vi "aft_Simulate_Edit_Template_(LMS).vi"(6 "State In":T2, 8 "error in":errorcluster, 11 "Diagram":T1) -> (0 "error out":errorcluster)   [LabVIEW 2017, in "NI_AdaptiveFilter.lvlib"]
uses:
  <vilib>/addons/Adaptive Filters/NI_AdaptiveFilter.lvlib
  <vilib>/addons/Adaptive Filters/Fixed-Point Simulation/LMS/AFT Simulate Fixed-Point FIR LMS.ctl
  <vilib>/XNodeSupport/XNodeTopLevelDiagramRef.ctl
  <vilib>/fxp/LVFixedPointOverflowPolicyTypeDef.ctl
  <vilib>/fxp/LVFixedPointQuantizationPolicyTypeDef.ctl
  <vilib>/addons/Adaptive Filters/Fixed-Point Simulation/LMS/AFT Simulate Fixed-Point FIR LMS.xnode
  <vilib>/XNodeSupport/NI_XNodeSupport.lvlib
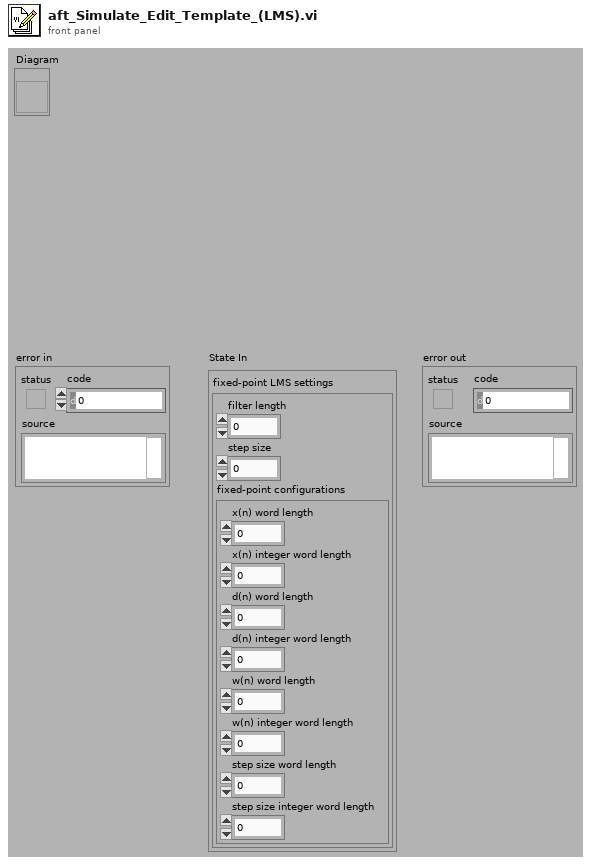
[diagram p1: front panel]
types:
  T1 = typedef "NI_XNodeSupport.lvlib/XNodeTopLevelDiagramRef.ctl" = refnum<vi>
  T2 = typedef "AFT Simulate Fixed-Point FIR LMS.xnode/AFT Simulate Fixed-Point FIR LMS.ctl" = cluster{"fixed-point LMS settings":cluster{"filter length":i32, "step size":dbl, "fixed-point configurations":cluster{"x(n) word length":i32, "x(n) integer word length":i32, "d(n) word length":i32, "d(n) integer word length":i32, "w(n) word length":i32, "w(n) integer word length":i32, "step size word length":i32, "step size integer word length":i32}}}
  T3 = typedef "LVFixedPointOverflowPolicyTypeDef.ctl" = enum32{"Wrap", "Saturate"}
  T4 = typedef "LVFixedPointQuantizationPolicyTypeDef.ctl" = enum32{"Truncate", "Round-Half-Up (Asymmetric)", "Round-Half-Even"}
  T5 = cluster{"filter length":i32, "step size":dbl, "fixed-point configurations":cluster{"x(n) word length":i32, "x(n) integer word length":i32, "d(n) word length":i32, "d(n) integer word length":i32, "w(n) word length":i32, "w(n) integer word length":i32, "step size word length":i32, "step size integer word length":i32}}
  T6 = cluster{"x(n) word length":i32, "x(n) integer word length":i32, "d(n) word length":i32, "d(n) integer word length":i32, "w(n) word length":i32, "w(n) integer word length":i32, "step size word length":i32, "step size integer word length":i32}
  T7 = typedef "LVFixedPointRepBitsTypeDef.ctl" = cluster{"Signed":bool, "Word Length":u32, "Integer Word Length":i32}
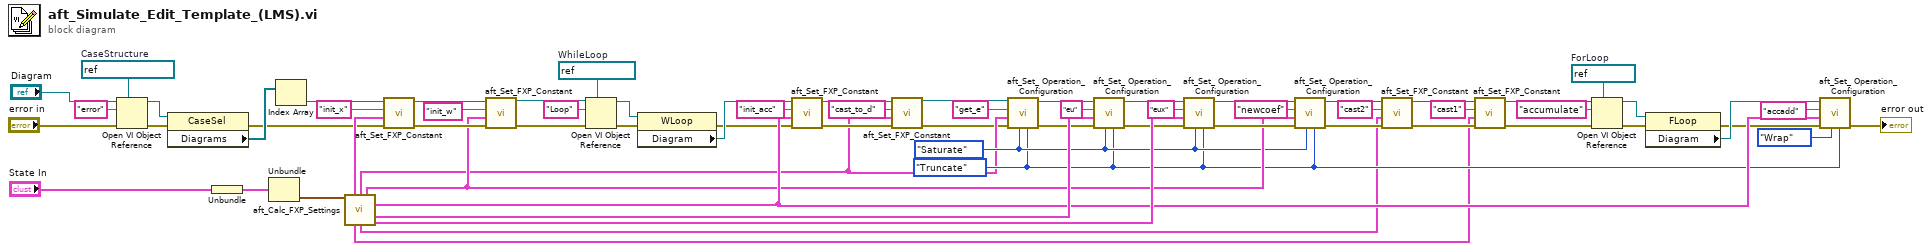
[diagram p0: block diagram]
diagram:
  w14 = LVFixedPointQuantizationPolicyTypeDef."Truncate" ("FXP Quantization Policy")
  w15 = LVFixedPointOverflowPolicyTypeDef."Saturate" ("FXP Overflow Policy")
  w43 = refnum<vi> refnum  # ForLoop
  w60 = refnum<vi> refnum  # WhileLoop
  w64 = refnum<vi> refnum  # CaseStructure
  n1 = Open VI Object Reference(7:w64, 8:"error in", 10:"error" ("name/order"), 11:"Diagram") -> (0:w19:errorcluster, 3:w58:refnum<vi>)
  n2 = property class="CaseSel"(reference=w58, error in=w19) -> (error out=w17:errorcluster, "Diagrams"=w62:refnum<vi>[])  [unwired: 1 out]
  n3 = Unbundle("State In") -> ("fixed-point LMS settings"=w66:T5)
  n4 = Unbundle(w66) -> ("fixed-point configurations"=w65:T6)  [unwired: 2 out]
  n5 = Index Array(array=w62) -> (element=w57:refnum<vi>)  [unwired: 1 in]
  n6 = call <vilib>:"aft_Calc_FXP_Settings.vi"("fixed-point configurations"=w65) -> ("x"=w27:T7, "d"=w12:T7, "w"=w20:T7, "init2"=w38:T7, "init3"=w49:T7, "cast 1"=w2:T7, "cast 2"=w1:T7, "init4"=w46:T7)  [unwired: 5 in, 2 out]
  n7 = call <vilib>:"aft_Set_FXP_Constant.vi"("error in (no error)"=w17, "fixed-point representation:bits"=w27, "name/order"="init_x", "diagram in"=w57) -> ("error out"=w25:errorcluster, "diagram out"=w23:refnum<vi>)  [unwired: 6 out]
  n8 = call <vilib>:"aft_Set_FXP_Constant.vi"("error in (no error)"=w25, "fixed-point representation:bits"=w20, "name/order"="init_w", "diagram in"=w23) -> ("error out"=w24:errorcluster, "diagram out"=w22:refnum<vi>)  [unwired: 6 out]
  n9 = Open VI Object Reference(7:w60, 8:w24, 10:"Loop" ("name/order"), 11:w22) -> (0:w37:errorcluster, 3:w56:refnum<vi>)
  n10 = property class="WLoop"(reference=w56, error in=w37) -> (error out=w36:errorcluster, "Diagram"=w54:refnum<vi>)  [unwired: 1 out]
  n11 = call <vilib>:"aft_Set_FXP_Constant.vi"("error in (no error)"=w36, "fixed-point representation:bits"=w38, "name/order"="init_acc", "diagram in"=w54) -> ("error out"=w28:errorcluster, "diagram out"=w29:refnum<vi>)  [unwired: 6 out]
  n12 = call <vilib>:"aft_Set_FXP_Constant.vi"("error in (no error)"=w28, "fixed-point representation:bits"=w12, "name/order"="cast_to_d", "diagram in"=w29) -> ("error out"=w10:errorcluster, "diagram out"=w11:refnum<vi>)  [unwired: 6 out]
  n13 = call <vilib>:"aft_Set_ Operation_Configuration.vi"("FXP Quantization Policy"=w14, "FXP Overflow Policy"=w15, "error in (no error)"=w10, "output type"=w12, "name/order"="get_e" ("name"), "diagram in"=w11) -> ("error out"=w35:errorcluster, "diagram out"=w50:refnum<vi>)  [unwired: 4 in]
  n14 = call <vilib>:"aft_Set_ Operation_Configuration.vi"("FXP Quantization Policy"=w14, "FXP Overflow Policy"=w15, "error in (no error)"=w35, "output type"=w49, "name/order"="eu" ("name"), "diagram in"=w50) -> ("error out"=w34:errorcluster, "diagram out"=w47:refnum<vi>)  [unwired: 4 in]
  n15 = call <vilib>:"aft_Set_ Operation_Configuration.vi"("FXP Quantization Policy"=w14, "FXP Overflow Policy"=w15, "error in (no error)"=w34, "output type"=w46, "name/order"="eux" ("name"), "diagram in"=w47) -> ("error out"=w33:errorcluster, "diagram out"=w44:refnum<vi>)  [unwired: 4 in]
  n16 = call <vilib>:"aft_Set_ Operation_Configuration.vi"("FXP Quantization Policy"=w14, "FXP Overflow Policy"=w15, "error in (no error)"=w33, "output type"=w20, "name/order"="newcoef" ("name"), "diagram in"=w44) -> ("error out"=w9:errorcluster, "diagram out"=w8:refnum<vi>)  [unwired: 4 in]
  n17 = call <vilib>:"aft_Set_FXP_Constant.vi"("error in (no error)"=w9, "fixed-point representation:bits"=w1, "name/order"="cast2", "diagram in"=w8) -> ("error out"=w6:errorcluster, "diagram out"=w5:refnum<vi>)  [unwired: 6 out]
  n18 = call <vilib>:"aft_Set_FXP_Constant.vi"("error in (no error)"=w6, "fixed-point representation:bits"=w2, "name/order"="cast1", "diagram in"=w5) -> ("error out"=w4:errorcluster, "diagram out"=w3:refnum<vi>)  [unwired: 6 out]
  n19 = Open VI Object Reference(7:w43, 8:w4, 10:"accumulate" ("name/order"), 11:w3) -> (0:w32:errorcluster, 3:w40:refnum<vi>)
  n20 = property class="FLoop"(reference=w40, error in=w32) -> (error out=w31:errorcluster, "Diagram"=w39:refnum<vi>)  [unwired: 1 out]
  n21 = call <vilib>:"aft_Set_ Operation_Configuration.vi"("FXP Quantization Policy"=w14, "FXP Overflow Policy"=LVFixedPointOverflowPolicyTypeDef."Wrap", "error in (no error)"=w31, "output type"=w38, "name/order"="accadd" ("name"), "diagram in"=w39) -> ("error out"=→"error out":errorcluster)  [unwired: 4 in, 1 out]
